vi "event.vi"() -> ()   [LabVIEW 2024]
panel:
  out "Output":string
  out "timeout":bool
  in  "stop":bool
  out "E":bool
  out "Q":bool
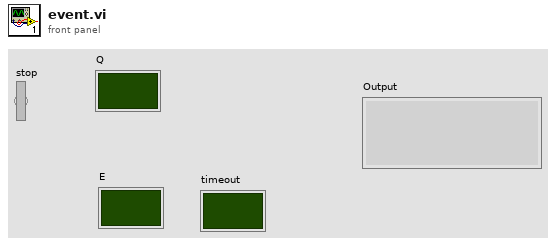
[diagram p1: front panel]
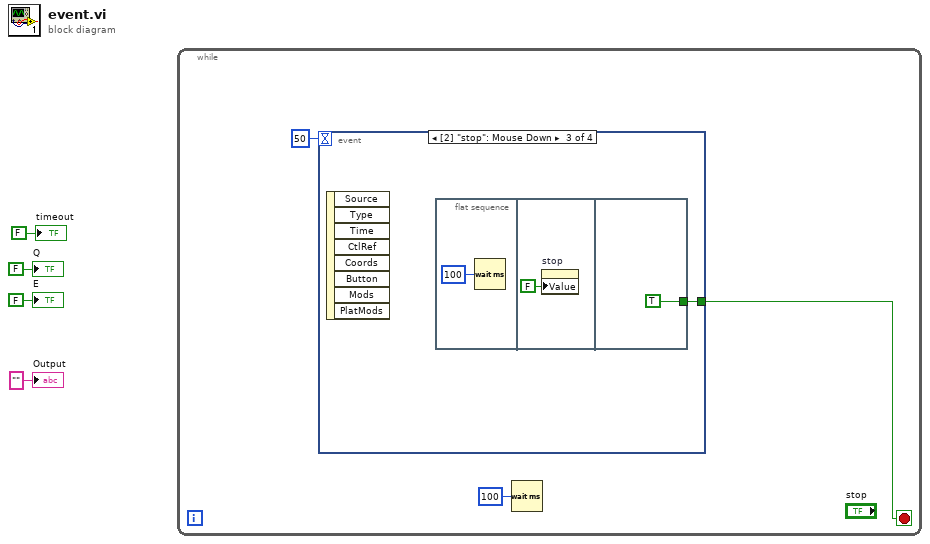
[diagram p0: block diagram]
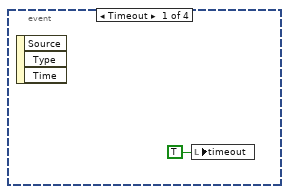
[diagram p2: hidden frame]
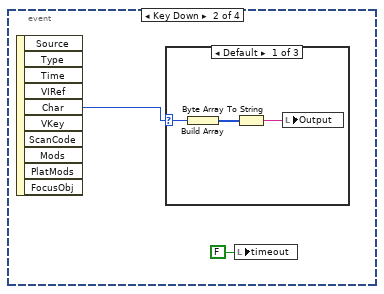
[diagram p3: hidden frame]
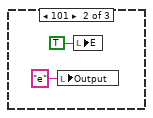
[diagram p4: hidden frame]
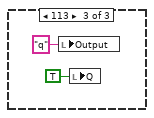
[diagram p5: hidden frame]
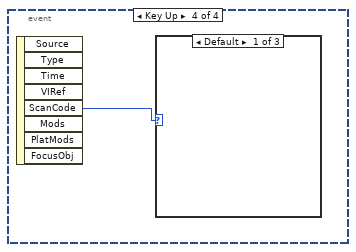
[diagram p6: hidden frame]
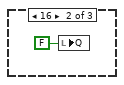
[diagram p7: hidden frame]
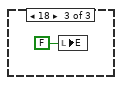
[diagram p8: hidden frame]
diagram:
  (unwired) FALSE ("Q")
  n1 = while {
    stop <- w5 stop-if-true
    n2 = event shown="[2] \"stop\": Mouse Down" {
      selector: _ -> [_ _ _ _]
      dyn-events: _ -> [_ _ _ _]
      timeout: 50 -> [_ _ _ _]
      tunnel: [_ _ w18 _] -> w5
      event Timeout {
        n3 = event-data() -> ()  [unwired: 1 in, 3 out]
        n4 = local write "timeout"(TRUE ("timeout")) -> ()
      }
      event Key Down {
        n5 = event-data() -> ("Char"=w10:i16)  [unwired: 1 in, 9 out]
        n6 = case shown="Default" w10 {
          selector: w10 -> [w13 _ _]
          frame Default {
            n7 = Build Array(w13) -> (w12:i16[])
            n8 = Byte Array To String(unsigned byte array=w12) -> (string=w11:string)
            n9 = local write "Output"(w11) -> ()
          }
          frame 101 {
            n10 = local write "Output"("e" ("Output")) -> ()
            n11 = local write "E"(TRUE ("E")) -> ()
          }
          frame 113 {
            n12 = local write "Output"("q" ("Output")) -> ()
            n13 = local write "Q"(TRUE ("Q")) -> ()
          }
        }
        n14 = local write "timeout"(FALSE ("timeout")) -> ()
      }
      event "stop": Mouse Down {
        n15 = event-data() -> ()  [unwired: 1 in, 8 out]
        n16 = flat-sequence {
          tunnel: [TRUE] -> w18
          frame #0 {
            n17 = Wait (ms)(milliseconds to wait=u32 100) -> ()  [unwired: 1 out]
          }
          frame #1 {
            n18 = property on="stop" class="Bool (strict)"("Value"=FALSE ("stop")) -> ()  [unwired: 2 in, 2 out]
          }
          frame #2 {
          }
        }
      }
      event Key Up {
        n19 = event-data() -> ("ScanCode"=w22:i16)  [unwired: 1 in, 7 out]
        n20 = case shown="Default" w22 {
          frame Default {
          }
          frame 16 {
            n21 = local write "Q"(FALSE ("Q")) -> ()
          }
          frame 18 {
            n22 = local write "E"(FALSE ("E")) -> ()
          }
        }
      }
    }
    n23 = Wait (ms)(milliseconds to wait=u32 100) -> ()  [unwired: 1 out]
  }
  "Q" <- FALSE ("Q")
  "E" <- FALSE ("E")
  "timeout" <- FALSE ("timeout")
  "Output" <- "" ("Output")
